vi "3D Coordinate Conversion.vi"   [LabVIEW 2010, in "NI_AALPro.lvlib"]
doc: "Converts coordinates between the Cartesian, spherical, and cylindrical coordinate systems. Wire data to the <B>Axis 1</B> input to determine the polymorphic instance to use or manually select the instance."
uses:
  NI_AALPro.lvlib
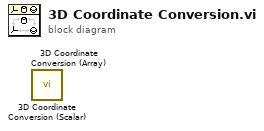
[diagram p0: block diagram]
diagram:
  n1 = call "3D Coordinate Conversion (Scalar).vi"() -> ()  [unwired: 8 in, 4 out]
  n2 = call "3D Coordinate Conversion (Array).vi"() -> ()  [unwired: 8 in, 4 out]
